vi "M01 TV.vi"(11 "NXT/EV3":T1) -> (3 "EV3 out":T1)   [LabVIEW 2016]
uses:
  <vilib>/NXT/Subs/LVHSConnector.ctl
  <vilib>/NXT/LegoClasses/BrickReference/BrickReference.lvclass
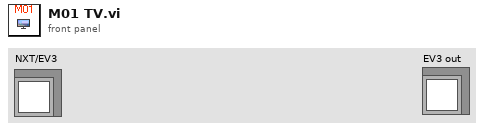
[diagram p1: front panel]
types:
  T1 = typedef "LVHSConnector.ctl" = refnum<class "BrickReference.lvclass">
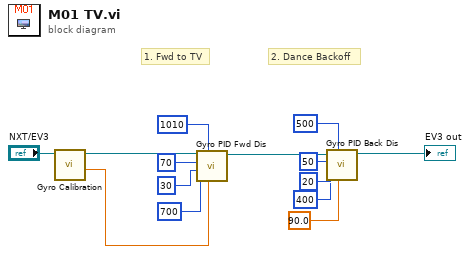
[diagram p0: block diagram]
diagram:
  # "2. Dance Backoff"
  # "1. Fwd to TV"
  n1 = call "Gyro Calibration.vi"("NXT/EV3"="NXT/EV3") -> ("Degrees"=w2:sgl, "NXT/EV3"=w4:T1)  [unwired: 6 in, 1 out]
  n2 = call "Gyro PID Fwd Dis.vi"("Target angle"=w2, "Threshold to stop"=1010, "Threshold to slow"=700, "Min. speed"=30, "Max. speed"=70, "EV3 in"=w4) -> ("EV3 out"=w9:T1)  [unwired: 5 in]
  n3 = call "Gyro PID Back Dis.vi"("Target angle"=sgl 90.0, "Threshold to stop"=500, "Threshold to slow"=400, "Min. speed"=20, "Max. speed"=50, "EV3 in"=w9) -> ("EV3 out"=→"EV3 out":T1)  [unwired: 5 in]
